vi "Filter Targets.vi"(1 "Targets In":T1[](array[typedef])) -> (0 "Targets Out":T1[](array[typedef]))   [LabVIEW 2009]
uses:
  Widget/Target.ctl
  Data Access Objects/Metadata/LBCB Number.ctl
  Data Access Objects/Metadata/Persistant DAO Actions.ctl
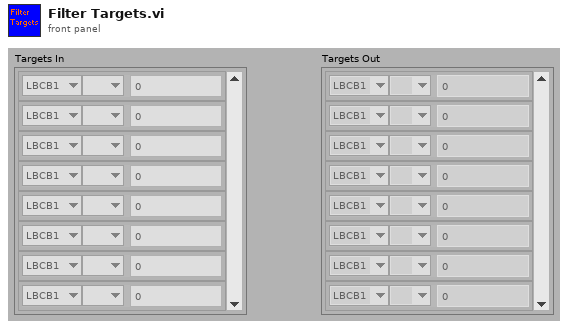
[diagram p1: front panel]
types:
  T1 = typedef "Target.ctl" = cluster{"LBCB Number":T2, "DOF Vectors":enum16{" ", "Dx", "Dy", "Dz", "Rx", "Ry", "Rz", "Fx", "Fy", "Fz", "Mx", "My", "Mz"}, "Amount":dbl}
  T2 = typedef "LBCB Number.ctl" = enum16{"LBCB1", "LBCB2"}
  T3 = typedef "Persistant DAO Actions.ctl" = enum16{"Init", "Get", "Set", "Load", "Save"}
  T4 = typedef "Number Of LBCBs.ctl" = enum16{"1", "2"}
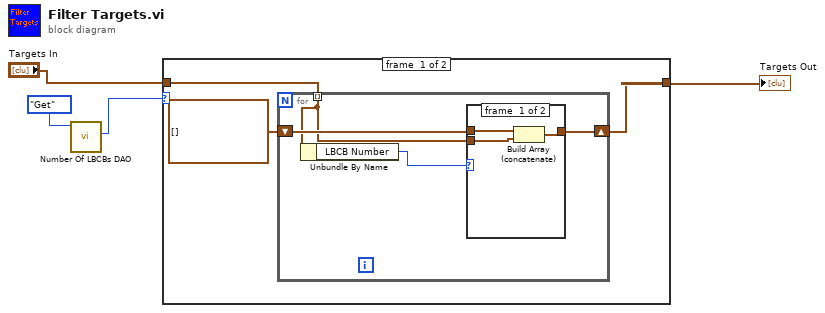
[diagram p0: block diagram]
diagram:
  n1 = call "Number Of LBCBs DAO.vi"("Actions"=Persistant_DAO_Actions."Get") -> ("Number of\nLBCBs Out"=w2:T4)  [unwired: 3 in, 7 out]
  n2 = case shown="\"1\"" w2 {
    tunnel: [w7 w16] -> w4
    tunnel: "Targets In" -> [w6 w16]
    frame #0 {
      n3 = for {
        shift-right: [w10] -> w7
        shift-left: T1[] [] -> [w11]
        tunnel: w6 -> [w9] mode=indexing
        n4 = Unbundle By Name(w9) -> ("LBCB Number"=w8:T2)
        n5 = case shown="\"LBCB1\"" w8 {
          tunnel: w11 -> [w13 w15]
          tunnel: [w14 w15] -> w10
          tunnel: w9 -> [w12 _]
          frame #0 {
            n6 = Build Array (concatenate)(w13, w12) -> (w14:T1[])
          }
          frame #1 {
          }
        }
      }
    }
    frame #1 {
    }
  }
  "Targets Out" <- w4
